vi "TipTilt Z.vi"() -> ()   [LabVIEW 2012]
uses:
  Madlib.dll
panel:
  out "Min. Z-Axis (um)":dbl format="%.4f"
  out "Max. Z-Axis (um)":dbl format="%.4f"
  out "Theta Y (mrad)":dbl format="%.4f"
  out "Theta X (mrad)":dbl format="%.4f"
  in  "Theta Y (mrad)":dbl format="%.4f"
  out "Center (um)":dbl format="%.4f"
  in  "Z-Axis (um)":dbl=50.0 format="%.4f"
  in  "Theta X (mrad)":dbl format="%.4f"
  out "Min. Theta Y (mrad)":dbl format="%.4f"
  out "Max. Theta Y (mrad)":dbl format="%.4f"
  out "Min. Theta X (mrad)":dbl format="%.4f"
  out "Max. Theta X (mrad)":dbl format="%.4f"
  out "Read Theta C (mrad)":dbl caption="C (um)" format="%.3f"
  out "Read Theta B (mrad)":dbl caption="B (um)" format="%.3f"
  out "Read Theta A (mrad)":dbl caption="A (um)" format="%.3f"
  in  "?":bool
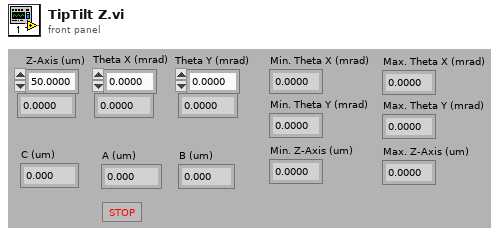
[diagram p1: front panel]
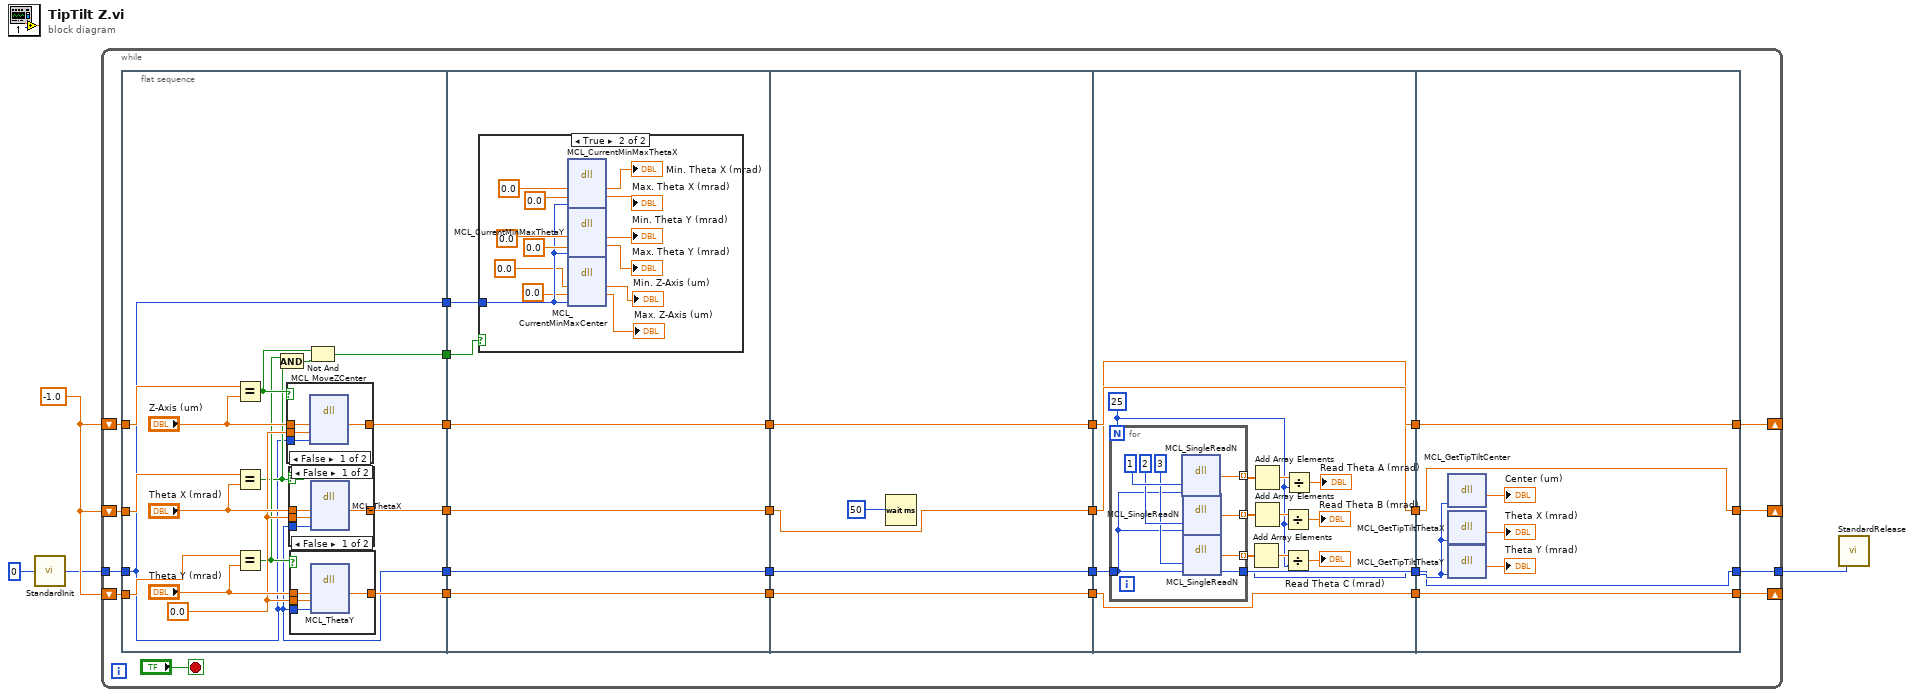
[diagram p0: block diagram]
diagram:
  w3 = -1.0
  n1 = call "StandardInit.vi"("Incoming Handle"=0) -> ("Outgoing Handle"=w2:i32)
  n2 = while {
    tunnel: w2 -> [w32]
    tunnel: [w31] -> w4
    shift-right: [w27] -> _
    shift-left: w3 -> [w26]
    shift-right: [w25] -> _
    shift-left: w3 -> [w24]
    shift-right: [w28] -> _
    shift-left: w3 -> [w29]
    stop <- "?" stop-if-true
    n3 = flat-sequence {
      tunnel: w32 -> [w33]
      tunnel: [w33] -> w23
      tunnel: w29 -> [w48]
      tunnel: [w46] -> w22
      tunnel: [w45] -> w21
      tunnel: w26 -> [w44]
      tunnel: [w42] -> w20
      tunnel: w24 -> [w41]
      tunnel: [w34] -> w6
      tunnel: [w33] -> w5
      tunnel: w23 -> [w69]
      tunnel: [w69] -> w19
      tunnel: w22 -> [w68]
      tunnel: [w68] -> w18
      tunnel: w21 -> [w67]
      tunnel: [w67] -> w17
      tunnel: w20 -> [w66]
      tunnel: [w66] -> w16
      tunnel: w6 -> [w65]
      tunnel: w5 -> [w64]
      tunnel: w19 -> [w86]
      tunnel: [w86] -> w15
      tunnel: w18 -> [w85]
      tunnel: [w85] -> w14
      tunnel: w17 -> [w84]
      tunnel: [w84] -> w13
      tunnel: w16 -> [w83]
      tunnel: [w83] -> w12
      tunnel: w15 -> [w102]
      tunnel: [w102] -> w11
      tunnel: [w101] -> w10
      tunnel: w14 -> [w90]
      tunnel: [w90] -> w9
      tunnel: w13 -> [w89]
      tunnel: [w89] -> w8
      tunnel: w12 -> [w88]
      tunnel: [w88] -> w7
      tunnel: w11 -> [w115]
      tunnel: [w114] -> w31
      tunnel: w10 -> [w114]
      tunnel: [w113] -> w28
      tunnel: w9 -> [w113]
      tunnel: [w112] -> w27
      tunnel: w8 -> [w112]
      tunnel: [w111] -> w25
      tunnel: w7 -> [w111]
      frame #0 {
        w39 = 0.0
        n4 = Equal?(x=w48, y="Z-Axis (um)") -> (x = y?=w38:bool)
        n5 = Equal?(x=w44, y="Theta X (mrad)") -> (x = y?=w36:bool)
        n6 = Equal?(x=w41, y="Theta Y (mrad)") -> (x = y?=w37:bool)
        n7 = And(x=w37, y=w36) -> (x .and. y?=w35:bool)
        n8 = case shown="False" w38 {
          tunnel: "Z-Axis (um)" -> [w62 w63]
          tunnel: [w61 w63] -> w46
          tunnel: w39 -> [w60 _]
          tunnel: w33 -> [w59 _]
          frame False {
            n9 = dll-call lib="C:/Users/Labview/Desktop/SRR/Madlib_x64/Labview Examples/MADLib.dll" fn="MCL_MoveZCenter"("center"=w62, "actual"=w60, "handle"=w59) -> ("center"=w61:dbl)  [unwired: 6 in, 2 out]
          }
          frame True {
          }
        }
        n10 = case shown="False" w36 {
          tunnel: [w57 w58] -> w45
          tunnel: "Theta X (mrad)" -> [w56 w58]
          tunnel: w39 -> [w55 _]
          tunnel: w33 -> [w54 _]
          frame False {
            n11 = dll-call lib="C:/Users/Labview/Desktop/SRR/Madlib_x64/Labview Examples/MADLib.dll" fn="MCL_ThetaX"("milliradians"=w56, "actual"=w55, "handle"=w54) -> ("milliradians"=w57:dbl)  [unwired: 6 in, 2 out]
          }
          frame True {
          }
        }
        n12 = case shown="False" w37 {
          tunnel: [w52 w53] -> w42
          tunnel: "Theta Y (mrad)" -> [w51 w53]
          tunnel: w39 -> [w50 _]
          tunnel: w33 -> [w49 _]
          frame False {
            n13 = dll-call lib="C:/Users/Labview/Desktop/SRR/Madlib_x64/Labview Examples/MADLib.dll" fn="MCL_ThetaY"("milliradians"=w51, "actual"=w50, "handle"=w49) -> ("milliradians"=w52:dbl)  [unwired: 6 in, 2 out]
          }
          frame True {
          }
        }
        n14 = Not And(1:w35, 2:w38) -> (0:w34:bool)
      }
      frame #1 {
        n15 = case shown="True" w65 {
          tunnel: w64 -> [_ w73]
          frame False {
          }
          frame True {
            n16 = dll-call lib="C:/Users/Labview/Desktop/SRR/Madlib_x64/Labview Examples/MADLib.dll" fn="MCL_CurrentMinMaxThetaX"("min"=0.0, "max"=0.0, "handle"=w73) -> ("min"=→"Min. Theta X (mrad)":dbl, "max"=→"Max. Theta X (mrad)":dbl)  [unwired: 5 in, 2 out]
            n17 = dll-call lib="C:/Users/Labview/Desktop/SRR/Madlib_x64/Labview Examples/MADLib.dll" fn="MCL_CurrentMinMaxThetaY"("min"=0.0, "max"=0.0, "handle"=w73) -> ("min"=→"Min. Theta Y (mrad)":dbl, "max"=→"Max. Theta Y (mrad)":dbl)  [unwired: 5 in, 2 out]
            n18 = dll-call lib="C:/Users/Labview/Desktop/SRR/Madlib_x64/Labview Examples/MADLib.dll" fn="MCL_CurrentMinMaxCenter"("min"=0.0, "max"=0.0, "handle"=w73) -> ("min"=→"Min. Z-Axis (um)":dbl, "max"=→"Max. Z-Axis (um)":dbl)  [unwired: 5 in, 2 out]
          }
        }
      }
      frame #2 {
        n19 = Wait (ms)(milliseconds to wait=50) -> ()  [unwired: 1 out]
      }
      frame #3 {
        w94 = 25
        n20 = for {
          N: w94 -> [_]
          tunnel: [w107] -> w98 mode=indexing
          tunnel: [w106] -> w100 mode=indexing
          tunnel: [w105] -> w99 mode=indexing
          tunnel: w102 -> [w104]
          tunnel: [w103] -> w101
          n21 = dll-call lib="C:/Users/Labview/Desktop/SRR/Madlib_x64/Labview Examples/MADLib.dll" fn="MCL_SingleReadN"("axis"=1, "handle"=w104) -> (w107:dbl)  [unwired: 5 in, 2 out]
          n22 = dll-call lib="C:/Users/Labview/Desktop/SRR/Madlib_x64/Labview Examples/MADLib.dll" fn="MCL_SingleReadN"("axis"=2, "handle"=w104) -> (w106:dbl)  [unwired: 5 in, 2 out]
          n23 = dll-call lib="C:/Users/Labview/Desktop/SRR/Madlib_x64/Labview Examples/MADLib.dll" fn="MCL_SingleReadN"("axis"=3, "handle"=w104) -> (w105:dbl, "handle"=w103:i32)  [unwired: 4 in, 2 out]
        }
        n24 = Add Array Elements(numeric array=w99) -> (sum=w95:dbl)
        n25 = Add Array Elements(numeric array=w98) -> (sum=w97:dbl)
        n26 = Add Array Elements(numeric array=w100) -> (sum=w96:dbl)
        n27 = Divide(x=w96, y=w94) -> (x/y=→"Read Theta B (mrad)":dbl)
        n28 = Divide(x=w95, y=w94) -> (x/y=→"Read Theta C (mrad)":dbl)
        n29 = Divide(x=w97, y=w94) -> (x/y=→"Read Theta A (mrad)":dbl)
      }
      frame #4 {
        n30 = dll-call lib="C:/Users/Labview/Desktop/SRR/Madlib_x64/Labview Examples/MADLib.dll" fn="MCL_GetTipTiltCenter"("handle"=w115) -> (→"Center (um)":dbl)  [unwired: 4 in, 2 out]
        n31 = dll-call lib="C:/Users/Labview/Desktop/SRR/Madlib_x64/Labview Examples/MADLib.dll" fn="MCL_GetTipTiltThetaX"("handle"=w115) -> (→"Theta X (mrad)":dbl)  [unwired: 4 in, 2 out]
        n32 = dll-call lib="C:/Users/Labview/Desktop/SRR/Madlib_x64/Labview Examples/MADLib.dll" fn="MCL_GetTipTiltThetaY"("handle"=w115) -> (→"Theta Y (mrad)":dbl)  [unwired: 4 in, 2 out]
      }
    }
  }
  n33 = call "StandardRelease.vi"("Outgoing Handle"=w4) -> ()  [unwired: 2 in]
